vi "Apply Module Configuration Data.vi"(8 "Error In":errorcluster, 11 "Compiled.Settings":T1 {"Configuration Data"."Properties"."U64 Properties"."UInt64 Write" format="%.0x"; "Configuration Data"."Properties"."U32 Properties"."UInt32 Write" format="%.0x"; "Configuration Data"."Properties"."Double Properties"."Double Write" format="%_20g"}) -> (0 "Error Out":errorcluster, 1 "Module Session Out":refnum<k21>, 2 "SLSC Module Name":refnum<k21>, 3 "Device Session":refnum<k21>)   [LabVIEW 2015, in "SLSC Module Template Engine.lvlib"]
uses:
  SLSC Module Template Engine.lvlib
  Shared/Compiled.Settings
  Shared/SLSC Dynamic Channel.ctl
  <vilib>/NI Veristand/Custom Device Tools/Custom Device Utility Library/Custom Device Utility Library.lvlib
  Shared/SLSC Module Template Shared.lvlib
  System Explorer/SLSC Module Template System Explorer.lvlib
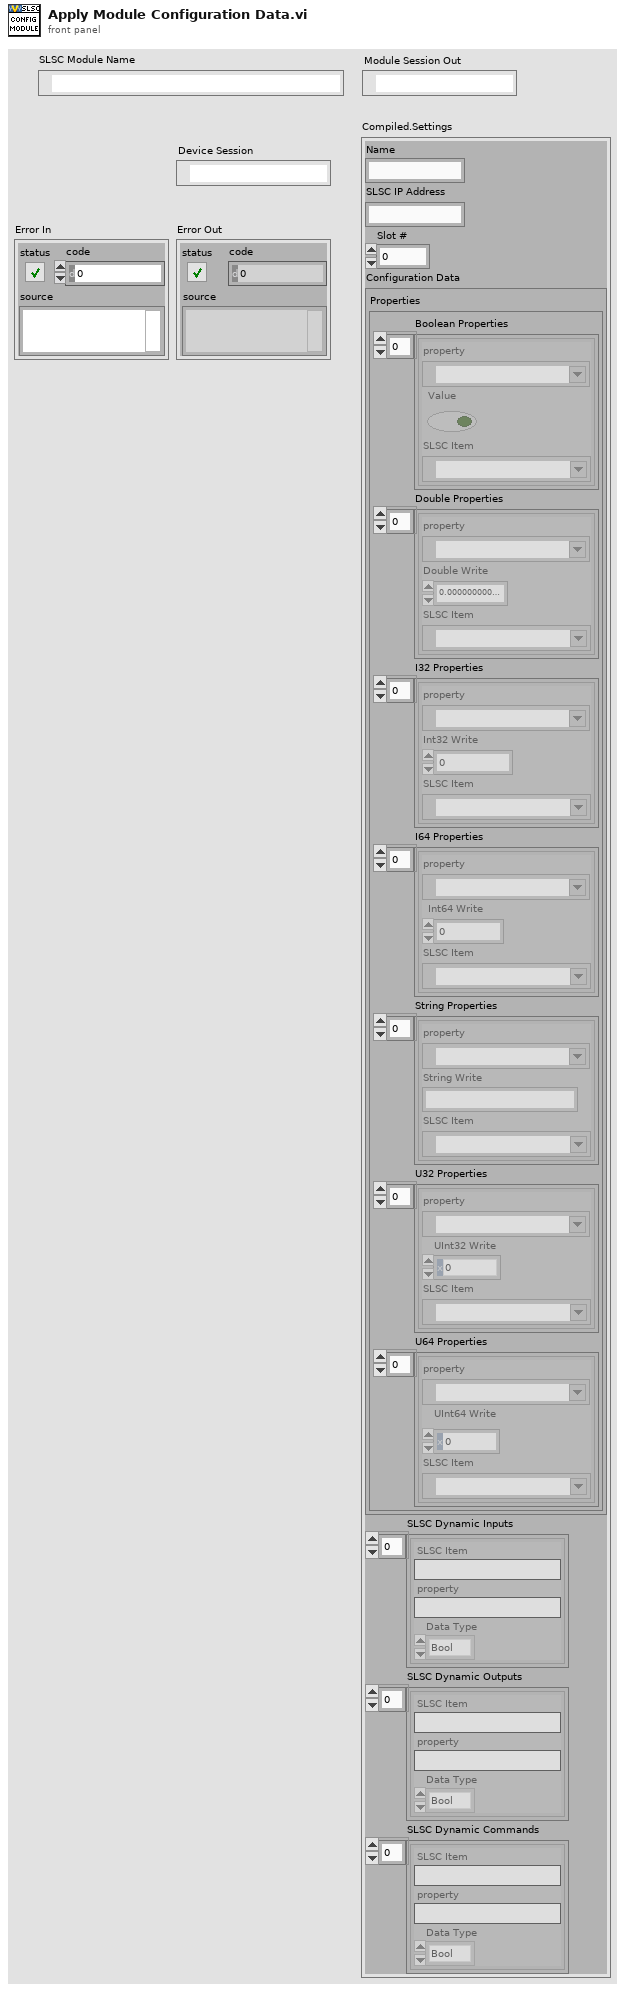
[diagram p1: front panel]
types:
  T1 = typedef "SLSC Module Template Shared.lvlib/Compiled.Settings" = cluster{"Name":string, "SLSC IP Address":string, "Slot #":i32, "Configuration Data":cluster{"Properties":cluster{"Boolean Properties":cluster{"property":refnum<k21>, "Value":bool, "SLSC Item":refnum<k21>}[], "Double Properties":cluster{"property":refnum<k21>, "Double Write":dbl, "SLSC Item":refnum<k21>}[], "I32 Properties":cluster{"property":refnum<k21>, "Int32 Write":i32, "SLSC Item":refnum<k21>}[], "I64 Properties":cluster{"property":refnum<k21>, "Int64 Write":i64, "SLSC Item":refnum<k21>}[], "String Properties":cluster{"property":refnum<k21>, "String Write":string, "SLSC Item":refnum<k21>}[], "U32 Properties":cluster{"property":refnum<k21>, "UInt32 Write":u32, "SLSC Item":refnum<k21>}[], "U64 Properties":cluster{"property":refnum<k21>, "UInt64 Write":u64, "SLSC Item":refnum<k21>}[]}}, "SLSC Dynamic Inputs":T2[], "SLSC Dynamic Outputs":T2[], "SLSC Dynamic Commands":T2[]}
  T2 = typedef "SLSC Module Template System Explorer.lvlib/SLSC Dynamic Channel.ctl" = cluster{"SLSC Item":string, "property":string, "Data Type":enum16{"Bool", "Double", "I32", "I64", "String", "U32", "U64"}}
  T3 = cluster{"Properties":cluster{"Boolean Properties":cluster{"property":refnum<k21>, "Value":bool, "SLSC Item":refnum<k21>}[], "Double Properties":cluster{"property":refnum<k21>, "Double Write":dbl, "SLSC Item":refnum<k21>}[], "I32 Properties":cluster{"property":refnum<k21>, "Int32 Write":i32, "SLSC Item":refnum<k21>}[], "I64 Properties":cluster{"property":refnum<k21>, "Int64 Write":i64, "SLSC Item":refnum<k21>}[], "String Properties":cluster{"property":refnum<k21>, "String Write":string, "SLSC Item":refnum<k21>}[], "U32 Properties":cluster{"property":refnum<k21>, "UInt32 Write":u32, "SLSC Item":refnum<k21>}[], "U64 Properties":cluster{"property":refnum<k21>, "UInt64 Write":u64, "SLSC Item":refnum<k21>}[]}}
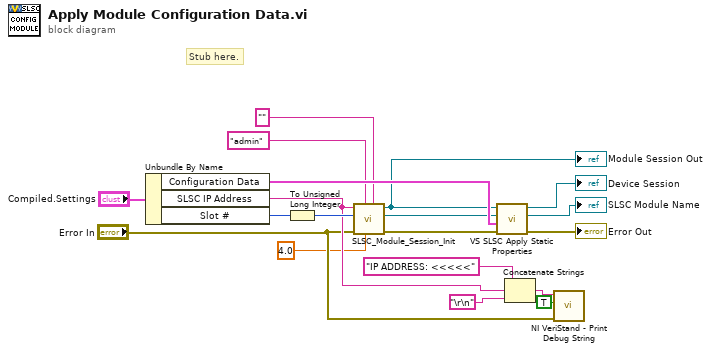
[diagram p0: block diagram]
diagram:
  # "Stub here."
  n1 = Unbundle By Name("Compiled.Settings") -> ("Configuration Data"=w18:T3, "SLSC IP Address"=w7:string, "Slot #"=w17:i32)
  n2 = To Unsigned Long Integer(number=w17) -> (unsigned 32bit integer=w16:u32)
  n3 = call "SLSC_Module_Session_Init.vi"("Password"="", "connect timeout (10 sec)"=4.0, "Username"="admin", "Error In"="Error In", "Slot #"=w16, "Chassis IP Address"=w7) -> ("Error Out"=w11:errorcluster, "SLSC Module Name"=w12:refnum<k21>, "Module Session Out"=w10:refnum<k21>)  [unwired: 2 in, 1 out]
  "Module Session Out" <- w10
  n4 = call "VS SLSC Apply Static Properties.vi"("error in (no error)"=w11, "Configuration Data"=w18, "SLSC Module Name in"=w12, "Refnum in"=w10) -> ("error out"=→"Error Out":errorcluster, "SLSC Module Name out"=→"SLSC Module Name":refnum<k21>, "Refnum out"=→"Device Session":refnum<k21>)  [unwired: 5 in]
  n5 = Concatenate Strings("IP ADDRESS: <<<<<" ("string"), w7, "\r\n") -> (w8:string)
  n6 = call <vilib>:"NI VeriStand - Print Debug String.vi"("error in (no error)"="Error In", "Add to log file? (T)"=TRUE, "Message"=w8) -> ()  [unwired: 8 in, 1 out]
